vi "Camera Begin.vi"(1 "Image Size":T1=enum."160x120") -> (0 "error out":errorcluster)   [LabVIEW 2012]
uses:
  <vilib>/Rock Robotics/WPI/Camera/WPI_CameraImageSize.ctl
  <vilib>/Rock Robotics/WPI/Camera/WPI_CameraWhite Balance Values.ctl
  <vilib>/Rock Robotics/WPI/Camera/WPI_CameraExposure Values.ctl
  <vilib>/Rock Robotics/WPI/Camera/WPI_CameraFrameRate.ctl
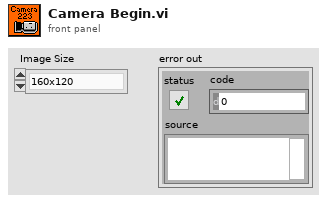
[diagram p1: front panel]
types:
  T1 = typedef "WPI_CameraImageSize.ctl" = enum16{"640x480", "320x240", "160x120"}
  T2 = typedef "WPI_CameraFrameRate.ctl" = u32
  T3 = typedef "WPI_CameraExposure Values.ctl" = enum16{"Auto", "Flicker-free 50 Hz", "Flicker-free 60 Hz", "Hold current"}
  T4 = typedef "WPI_CameraWhite Balance Values.ctl" = enum16{"Auto", "Fixed indoor", "Fixed outdoor 1", "Fixed outdoor 2", "Fixed fluorescent 1", "Fixed fluorescent 2", "Hold current"}
  T5 = typedef "WPI_CameraDevRef.ctl" = cluster{"Camera Address":string, "CameraStatus":errorcluster, "Acquire Image Notifier":refnum<notifier>}
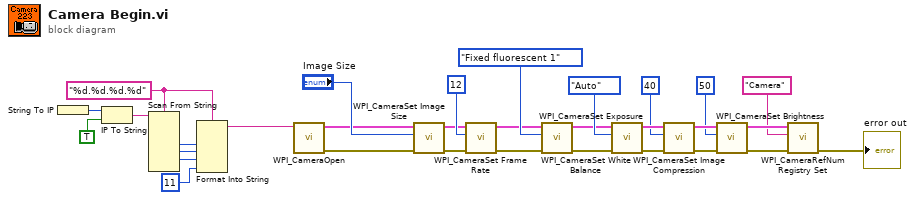
[diagram p0: block diagram]
diagram:
  w29 = "%d.%d.%d.%d" ("format string")
  n1 = String To IP() -> (0:w22:u32)  [unwired: 1 in]
  n2 = IP To String(1:TRUE ("dot notation? (F)"), 2:w22) -> (0:w24:string)
  n3 = Scan From String(format string=w29, input string=w24) -> (output 1=w25:i32, output 2=w26:i32, output 3=w27:i32)  [unwired: 7 in, 3 out]
  n4 = Format Into String(format string=w29, w25, w26, w27, 11 ("Compression")) -> (resulting string=w30:string)  [unwired: 2 in, 1 out]
  n5 = call <vilib>:"WPI_CameraOpen.vi"("Camera Address"=w30) -> ("error out"=w10:errorcluster, "CameraDevRef"=w9:T5)  [unwired: 1 in, 8 out]
  n6 = call <vilib>:"WPI_CameraSet Image Size.vi"("error in (no error)"=w10, "Image Size"="Image Size", "CameraDevRef"=w9) -> ("error out"=w11:errorcluster, "CameraDevRef Out"=w8:T5)  [unwired: 7 out]
  n7 = call <vilib>:"WPI_CameraSet Frame Rate.vi"("error in (no error)"=w11, "Frame Rate (fps)"=T2 12, "CameraDevRef"=w8) -> ("error out"=w12:errorcluster, "CameraDevRef Out"=w6:T5)  [unwired: 7 out]
  n8 = call <vilib>:"WPI_CameraSet White Balance.vi"("error in (no error)"=w12, "White Balance"=WPI_CameraWhite_Balance_Values."Fixed fluorescent 1", "CameraDevRef"=w6) -> ("error out"=w13:errorcluster, "CameraDevRef Out"=w7:T5)  [unwired: 7 out]
  n9 = call <vilib>:"WPI_CameraSet Exposure.vi"("error in (no error)"=w13, "Exposure"=WPI_CameraExposure_Values."Auto", "CameraDevRef"=w7) -> ("error out"=w14:errorcluster, "CameraDevRef Out"=w4:T5)  [unwired: 7 out]
  n10 = call <vilib>:"WPI_CameraSet Image Compression.vi"("error in (no error)"=w14, "Compression"=40, "CameraDevRef"=w4) -> ("error out"=w15:errorcluster, "CameraDevRef Out"=w5:T5)  [unwired: 7 out]
  n11 = call <vilib>:"WPI_CameraSet Brightness.vi"("error in (no error)"=w15, "Brightness"=50, "CameraDevRef"=w5) -> ("error out"=w17:errorcluster, "CameraDevRef Out"=w16:T5)  [unwired: 7 out]
  n12 = call <vilib>:"WPI_CameraRefNum Registry Set.vi"("error in (no error)"=w17, "refnum name"="Camera", "CameraDevRef"=w16) -> ("error out"=→"error out":errorcluster)  [unwired: 8 out]
